vi "SubVi_Duracion.vi"(0 "Tiempo 2":string="08:28:19 a. m.") -> (7 "Tiempo string":string, 8 "Duracion String":string, 9 "Duracion":i32)   [LabVIEW 2017]
panel:
  out "Hora 2":string
  out "Minutos 2":string
  out "Segundos 2":string
  out "time string 2":string
  out "Hora Numerica 2":i32
  out "Minutos Numericos 2":i32
  out "Segundos Numericos 2":i32
  out "Tiempo 2":string
  out "Segundos Totales 2":i32
  out "Segundos Totales":i32
  out "Tiempo":string
  out "Segundos Numericos":i32
  out "Minutos Numericos":i32
  out "Hora Numerica":i32
  out "Segundos":string
  out "Minutos":string
  out "Hora":string
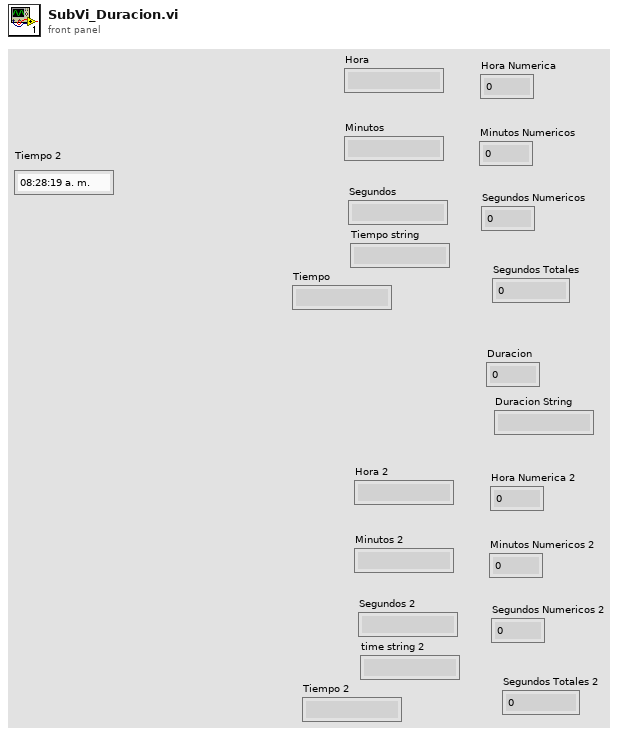
[diagram p1: front panel]
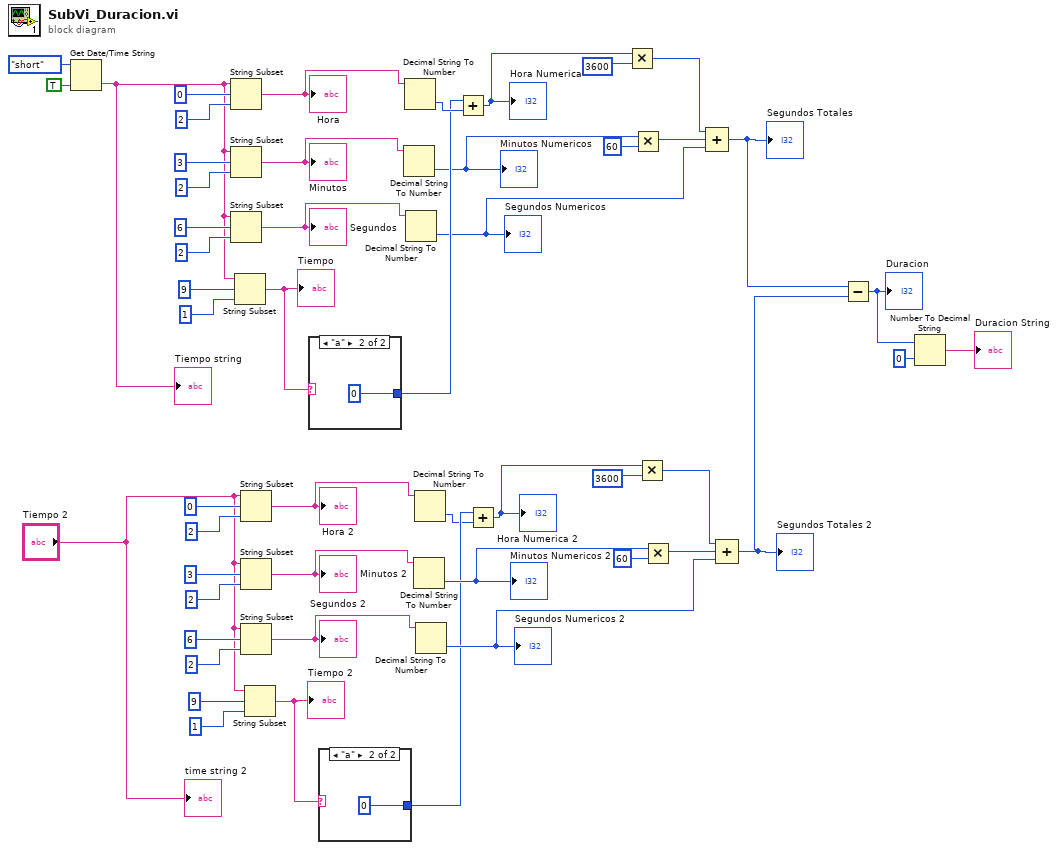
[diagram p0: block diagram]
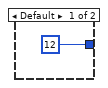
[diagram p2: hidden frame]
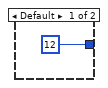
[diagram p3: hidden frame]
diagram:
  n1 = Get Date/Time String(date format (0)=enum16{"short", "long", "abbreviated"}."short", want seconds? (F)=TRUE) -> (time string=w38:string)  [unwired: 1 in, 1 out]
  "Tiempo string" <- w38
  n2 = String Subset(string=w38, offset (0)=0, length (rest)=2 ("length (rest)")) -> (substring=w43:string)
  "Hora" <- w43
  n3 = String Subset(string=w38, offset (0)=3, length (rest)=2 ("length (rest)")) -> (substring=w42:string)
  "Minutos" <- w42
  n4 = String Subset(string=w38, offset (0)=6, length (rest)=2 ("length (rest)")) -> (substring=w41:string)
  "Segundos" <- w41
  n5 = String Subset(string=w38, offset (0)=9, length (rest)=1 ("length (rest)")) -> (substring=w37:string)
  "Tiempo" <- w37
  n6 = String Subset(string="Tiempo 2", offset (0)=0, length (rest)=2 ("length (rest)")) -> (substring=w13:string)
  "Hora 2" <- w13
  n7 = String Subset(string="Tiempo 2", offset (0)=3, length (rest)=2 ("length (rest)")) -> (substring=w14:string)
  "Minutos 2" <- w14
  n8 = String Subset(string="Tiempo 2", offset (0)=6, length (rest)=2 ("length (rest)")) -> (substring=w15:string)
  "Segundos 2" <- w15
  n9 = String Subset(string="Tiempo 2", offset (0)=9, length (rest)=1 ("length (rest)")) -> (substring=w18:string)
  "Tiempo 2" <- w18
  n10 = case shown="\"a\"" w37 {
    tunnel: [12 0] -> w35
    frame Default {
    }
    frame "a" {
    }
  }
  n11 = case shown="\"a\"" w18 {
    tunnel: [12 0] -> w20
    frame Default {
    }
    frame "a" {
    }
  }
  n12 = Decimal String To Number(string=w42) -> (number=w33:i32)  [unwired: 2 in, 1 out]
  "Minutos Numericos" <- w33
  n13 = Decimal String To Number(string=w43) -> (number=w36:i32)  [unwired: 2 in, 1 out]
  n14 = Decimal String To Number(string=w41) -> (number=w29:i32)  [unwired: 2 in, 1 out]
  "Segundos Numericos" <- w29
  n15 = Decimal String To Number(string=w14) -> (number=w22:i32)  [unwired: 2 in, 1 out]
  "Minutos Numericos 2" <- w22
  n16 = Decimal String To Number(string=w13) -> (number=w19:i32)  [unwired: 2 in, 1 out]
  n17 = Decimal String To Number(string=w15) -> (number=w26:i32)  [unwired: 2 in, 1 out]
  "Segundos Numericos 2" <- w26
  n18 = Add(x=w35, y=w36) -> (x+y=w28:i32)
  "Hora Numerica" <- w28
  n19 = Add(x=w20, y=w19) -> (x+y=w27:i32)
  "Hora Numerica 2" <- w27
  n20 = Multiply(x=w28, y=3600) -> (x*y=w31:i32)
  n21 = Multiply(x=w33, y=60) -> (x*y=w30:i32)
  n22 = Multiply(x=w27, y=3600) -> (x*y=w24:i32)
  n23 = Multiply(x=w22, y=60) -> (x*y=w25:i32)
  n24 = Compound Arithmetic op=ADD(w31, w30, w29) -> (w5:i32)
  "Segundos Totales" <- w5
  n25 = Compound Arithmetic op=ADD(w24, w25, w26) -> (w4:i32)
  "Segundos Totales 2" <- w4
  n26 = Subtract(x=w5, y=w4) -> (x-y=w3:i32)
  "Duracion" <- w3
  n27 = Number To Decimal String(number=w3, width (-)=i16 0) -> (decimal integer string=→"Duracion String":string)
  "time string 2" <- "Tiempo 2"
